vi "Init.vi"(8 "error in (no error)":errorcluster, 9 "I2C Chanel(1)":i32=1, 10 "I2C Slave Address (61)":u16=61, 11 "LINX Resource":T1) -> (0 "error out":errorcluster, 3 "PCA out":refnum<class "PCA.lvclass">)   [LabVIEW 2022 SP3, in "PCA9685.lvlib" / "PCA.lvclass"]
uses:
  PCA.lvclass
  <vilib>/MakerHub/LINX/Private/Type Defs/LINX Ref.ctl
  <vilib>/MakerHub/LINX/Private/Type Defs/Platform.ctl
  <vilib>/MakerHub/LINX/Private/Type Defs/Interface.ctl
  <vilib>/MakerHub/LINX/Private/Device/Type Defs/LINX Device Config.ctl
  <vilib>/MakerHub/LINX/Private/Device/Type Defs/TCP Config.ctl
  <vilib>/MakerHub/LINX/Private/Device/Type Defs/Channels.ctl
  typedefs/LinxI2C.ctl
  PCA.lvclass/PCA.ctl
  <vilib>/MakerHub/LINX/LMH-LINX.lvlib
  <vilib>/MakerHub/LINX/Private/Device/Device.lvlib
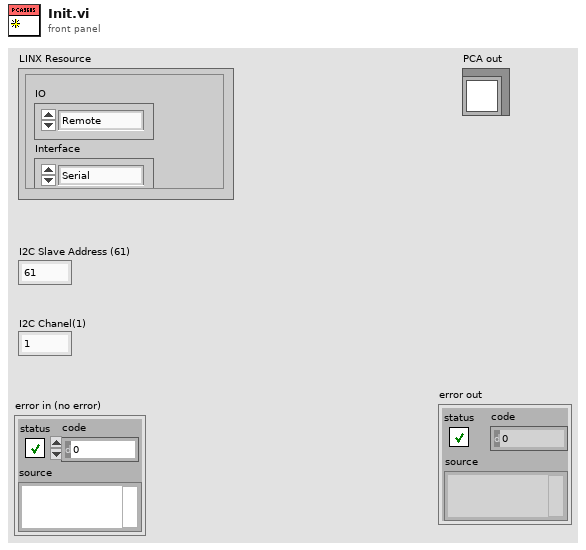
[diagram p1: front panel]
types:
  T1 = typedef "LMH-LINX.lvlib/LINX Ref.ctl" = cluster{"IO":T2, "Interface":T3, "LINX Device Config":T4}
  T2 = typedef "LMH-LINX.lvlib/Platform.ctl" = enum16{"Remote", "Local"}
  T3 = typedef "LMH-LINX.lvlib/Interface.ctl" = enum16{"Serial", "TCP"}
  T4 = typedef "LMH-LINX.lvlib/Device.lvlib/LINX Device Config.ctl" = cluster{"Interface":T3, "COM Port":refnum<visa-resource-name>, "TCP Configuration":T5, "Device Family":u8, "Device ID":u8, "Device Name":string, "TCP Ref":refnum<k5>, "Channels":T6}
  T5 = typedef "LMH-LINX.lvlib/Device.lvlib/TCP Config.ctl" = cluster{"IP Address":string, "Port":u16}
  T6 = typedef "LMH-LINX.lvlib/Channels.ctl" = cluster{"DI":u8[], "DO":u8[], "AI":u8[], "AO":u8[], "PWM":u8[], "QE":u8[], "UART":u8[], "I2C 2":u8[], "SPI":u8[], "CAN":u8[], "Servo":u8[], "AI Ref (V)":dbl, "AI Resolution (Bits)":u8, "AO Ref (V)":dbl, "AO Resolution (Bits)":u8}
  T7 = typedef "PCA9685.lvlib/PCA.lvclass/LinxI2C.ctl" = cluster{"I2C Slave Address (0)":u16, "I2C Chanel":u16, "LINX Resource":T1}
  T8 = typedef "PCA9685.lvlib/PCA.lvclass/Led.ctl" = cluster{"Led_onL":i8, "Led_onH":i8, "Led_offL":i8, "Led_offH":i8}
  T9 = typedef "PCA9685.lvlib/PCA.lvclass/Mode1.ctl" = cluster{"Allcall":u8, "sub3":u8, "sub2":u8, "Sleep":u8, "sub1":u8, "AutoInkrement":u8, "Restart":u8, "EXTclk":u8}
  T10 = typedef "PCA9685.lvlib/PCA.lvclass/Mode2.ctl" = cluster{"Outne_0":u8, "Outne_1":u8, "Outdrv":u8, "invrt":u8, "Och":u8}
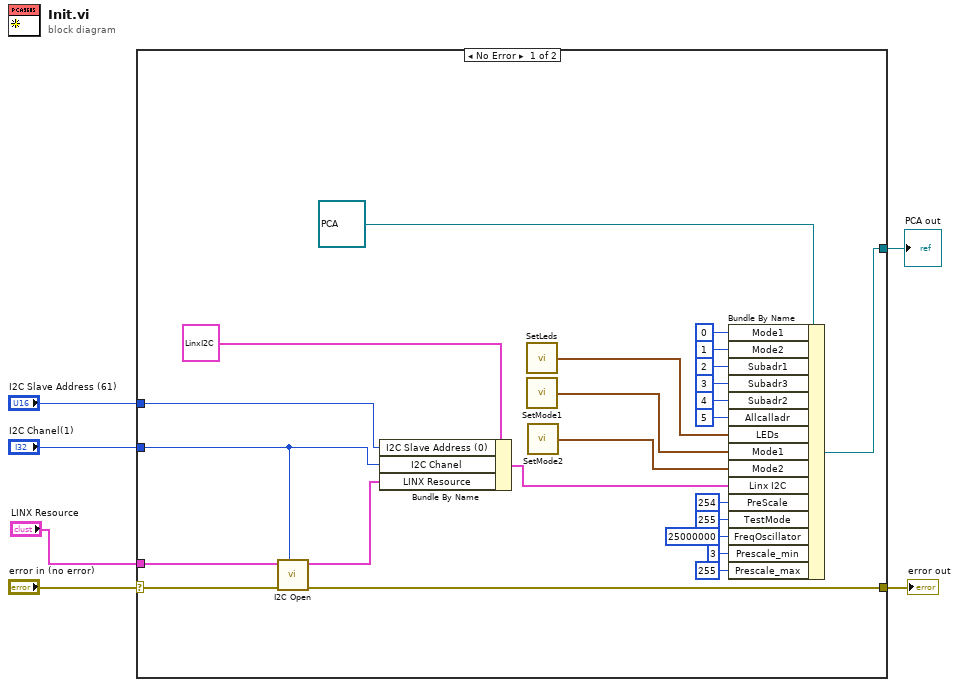
[diagram p0: block diagram]
diagram:
  n1 = case shown="No Error" "error in (no error)" {
    selector: "error in (no error)" -> [w10 w31]
    tunnel: [w9 w31] -> w5
    tunnel: [w30 _] -> w1
    tunnel: "I2C Slave Address (61)" -> [w13 _]
    tunnel: "I2C Chanel(1)" -> [w8 _]
    tunnel: "LINX Resource" -> [w12 _]
    frame No Error {
      n2 = call <vilib>:"I2C Open.vi"("I2C Channel (0)"=w8, "Error In"=w10, "LINX Resource"=w12) -> ("Error Out"=w9:errorcluster, "LINX Resource"=w11:T1)  [unwired: 7 in]
      n3 = Bundle By Name(cluster=T7 {"I2C Slave Address (0)"=0, "I2C Chanel"=0, "LINX Resource"={"IO"=enum."Remote", "Interface"=enum."Serial", "LINX Device Config"={"Interface"=enum."Serial", "COM Port"="COM13", "TCP Configuration"={"IP Address"="", "Port"=0}, "Device Family"=1, "Device ID"=1, "Device Name"="myRIO-1900", "TCP Ref"=refnum, "Channels"={"DI"=[0, 1, 2, 3, 4, 5, 6, 7, 8, 9, 10, 11, 12, 13, 14, 15, 16, 17, 18, 19, 20, 21, 22, 23, 24, 25, 26, 27, 28, 29, 30, 31, 32, 33, 34, 35, 36, 37, 38, 39, 40, 41, 42, 43, 44, 45, 46], "DO"=[0, 1, 2, 3, 4, 5, 6, 7, 8, 9, 10, 11, 12, 13, 14, 15, 16, 17, 18, 19, 20, 21, 22, 23, 24, 25, 26, 27, 28, 29, 30, 31, 32, 33, 34, 35, 36, 37, 38, 39, 40, 41, 42, 43, 44, 45, 46], "AI"=[0, 1, 2, 3, 4, 5, 6, 7, 8, 9, 10, 11], "AO"=[], "PWM"=[3, 5, 6, 9, 10], "QE"=[], "UART"=[0, 1], "I2C 2"=[0], "SPI"=[0], "CAN"=[], "Servo"=[], "AI Ref (V)"=0.0, "AI Resolution (Bits)"=0, "AO Ref (V)"=0.0, "AO Resolution (Bits)"=0}}}} ("Linx I2C"), "I2C Slave Address (0)"=w13, "I2C Chanel"=w8, "LINX Resource"=w11) -> (w14:T7)
      n4 = call "SetLeds.vi"() -> ("Array"=w23:T8[])  [unwired: 1 in]
      n5 = call "SetMode1.vi"() -> ("output cluster"=w22:T9)  [unwired: 1 in]
      n6 = call "SetMode2.vi"() -> ("output cluster"=w21:T10)  [unwired: 1 in]
      n7 = Bundle By Name(cluster=refnum<class "PCA.lvclass"> refnum ("PCA out"), "Mode1"=u8 0, "Mode2"=u8 1 ("Mode1"), "Subadr1"=u8 2 ("Mode1"), "Subadr3"=u8 3 ("Mode1"), "Subadr2"=u8 4 ("Mode1"), "Allcalladr"=u8 5 ("Mode1"), "LEDs"=w23, "Mode1"=w22, "Mode2"=w21, "Linx I2C"=w14, "PreScale"=u8 254, "TestMode"=u8 255 ("PreScale"), "FreqOscillator"=u32 25000000, "Prescale_min"=u32 3, "Prescale_max"=u32 255) -> (w30:refnum<class "PCA.lvclass">)
    }
    frame Error {
    }
  }
  "error out" <- w5
  "PCA out" <- w1
